vi "save rtos distribution.vi"() -> ()   [LabVIEW 2020]
uses:
  <vilib>/Utility/file.llb/Write Delimited Spreadsheet (I64).vi
panel:
  in  "timing data out":path
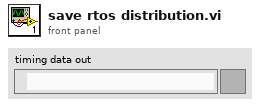
[diagram p1: front panel]
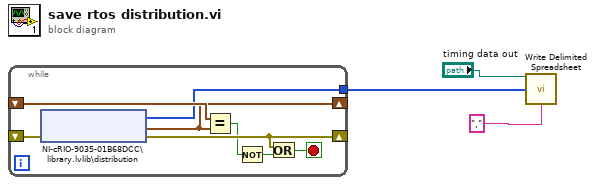
[diagram p0: block diagram]
diagram:
  n1 = while {
    shift-right: [w4] -> _
    shift-left: _ -> [w10]
    shift-right: [w9] -> _
    shift-left: _ -> [w11]
    tunnel: [w6] -> w1
    stop <- w5 stop-if-true
    n2 = shared-variable "NI-cRIO-9035-01B68DCC\\library.lvlib\\distribution"(error in=w11) -> (w6:i32[], error out=w9:errorcluster, w4:timestamp)
    n3 = Equal?(x=w10, y=w4) -> (x = y?=w7:bool)
    n4 = Not(x=w7) -> (.not. x?=w8:bool)
    n5 = Or(x=w9, y=w8) -> (x .or. y?=w5:bool)
  }
  n6 = call-poly <vilib>:"Write Delimited Spreadsheet.vi"("file path (dialog if empty)"="timing data out", "1D data"=w1, "delimiter (\\t)"=",") -> ()  [unwired: 11 in, 2 out]
